vi "young_dataparse.vi"(6 "Current Time":timestamp, 8 "Tips In":i32, 9 "TB In":i32, 11 "Poll Response":string) -> (0 "Tips Out":i32, 1 "TB Out":i32, 2 "Output Array":dbl[](array[numeric]))   [LabVIEW 2018]
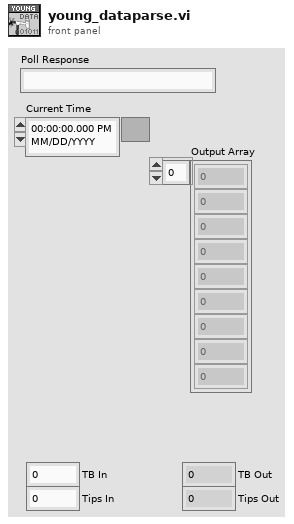
[diagram p1: front panel]
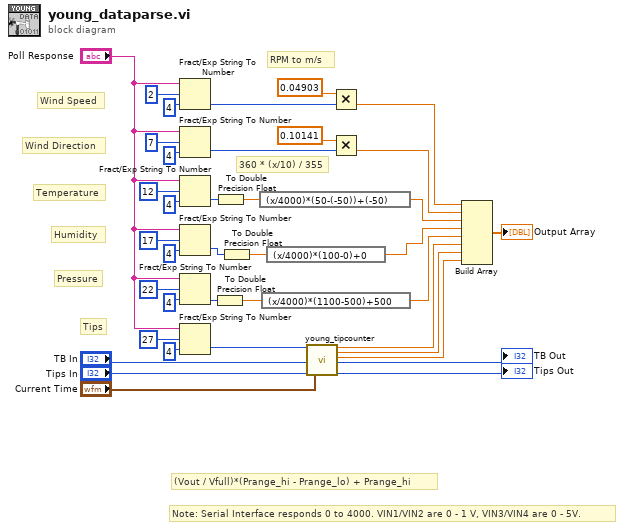
[diagram p0: block diagram]
diagram:
  # "360 * (x/10) / 355"
  # "RPM to m/s"
  # "Note: Serial Interface responds 0 to 4000. VIN1/VIN2 are 0 - 1 V, VIN3/VIN4 are 0 - 5V."
  # "(Vout / Vfull)*(Prange_hi - Prange_lo) + Prange_hi"
  # "Tips"
  # "Wind Direction"
  # "Wind Speed"
  # "Pressure"
  # "Humidity"
  # "Temperature"
  n1 = Fract/Exp String To Number(string="Poll Response", offset=2 ("offset (0)"), default (0 dbl)=4 ("length (rest)")) -> (number=w28:i32)  [unwired: 1 in, 1 out]
  n2 = Fract/Exp String To Number(string="Poll Response", offset=7 ("offset (0)"), default (0 dbl)=4 ("offset (0)")) -> (number=w27:i32)  [unwired: 1 in, 1 out]
  n3 = Fract/Exp String To Number(string="Poll Response", offset=12 ("offset (0)"), default (0 dbl)=4 ("offset (0)")) -> (number=w6:i32)  [unwired: 1 in, 1 out]
  n4 = Fract/Exp String To Number(string="Poll Response", offset=17 ("offset (0)"), default (0 dbl)=4 ("offset (0)")) -> (number=w3:i32)  [unwired: 1 in, 1 out]
  n5 = Fract/Exp String To Number(string="Poll Response", offset=22 ("offset (0)"), default (0 dbl)=4 ("offset (0)")) -> (number=w8:i32)  [unwired: 1 in, 1 out]
  n6 = Fract/Exp String To Number(string="Poll Response", offset=27 ("offset (0)"), default (0 dbl)=4 ("offset (0)")) -> (number=w11:i32)  [unwired: 1 in, 1 out]
  n7 = To Double Precision Float(number=w8) -> (double precision float=w7:dbl)
  n8 = To Double Precision Float(number=w6) -> (double precision float=w5:dbl)
  n9 = To Double Precision Float(number=w3) -> (double precision float=w2:dbl)
  n10 = expression code="(x/4000)*(50-(-50))+(-50)"(w5) -> (w4:dbl)
  n11 = expression code="(x/4000)*(1100-500)+500"(w7) -> (w9:dbl)
  n12 = expression code="(x/4000)*(100-0)+0"(w2) -> (w1:dbl)
  n13 = call "young_tipcounter.vi"("Poll Response (TB Count)"=w11, "TB In"="TB In", "Tips In"="Tips In", "Current Time"="Current Time") -> ("Cumulative Tip Count"=w19:dbl, "Rain Rate"=w17:dbl, "Cumulative Rain Fall"=w18:dbl, "TB Out"=→"TB Out":i32, "Tips Out"=→"Tips Out":i32)  [unwired: 11 in]
  n14 = Multiply(x=0.04903, y=w28) -> (x*y=w22:dbl)
  n15 = Multiply(x=0.10141, y=w27) -> (x*y=w21:dbl)
  n16 = Build Array(w22, w21, w4, w1, w9, w19, w17, w18) -> (→"Output Array":dbl[])
